vi "Set DDS Trigger Source Enge.vi"(8 "error in (no error)":errorcluster, 10 "enge":u32, 11 "channel_index":u8) -> (0 "error out":errorcluster)   [LabVIEW 2021, in "vmmso.lvlib"]
doc: "DLL_API void WINAPI SetDDSTriggerSourceEnge(unsigned char channel_index, unsigned int enge);"
uses:
  vmmso.lvlib
  vmmso.dll
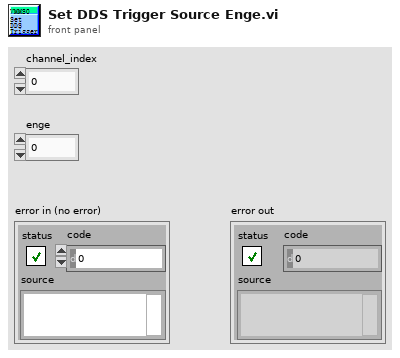
[diagram p1: front panel]
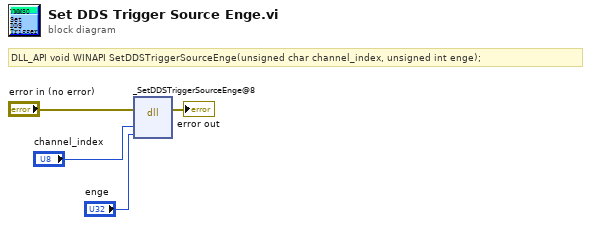
[diagram p0: block diagram]
diagram:
  # "DLL_API void WINAPI SetDDSTriggerSourceEnge(unsigned char channel_index, unsigned int enge);"
  n1 = dll-call lib="O:/MSO/library/demo-Labview/vmmso/vmmso.*" fn="_SetDDSTriggerSourceEnge@8"(error in="error in (no error)", "channel_index"="channel_index", "enge"="enge") -> (error out=→"error out":errorcluster)  [unwired: 5 in, 1 out]
